vi "UP-COUNTER-V2.vi"() -> (3 "COMPARATOR INPUT 1":u32)   [LabVIEW 2016]
panel:
  in  "LOWER LIMIT":u32=22
  in  "UPPER LIMIT":u32=26
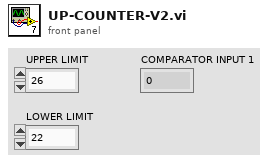
[diagram p1: front panel]
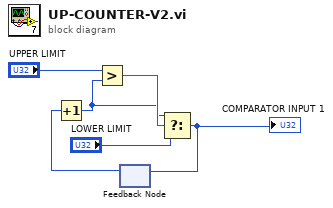
[diagram p0: block diagram]
diagram:
  n1 = feedback #1() -> (w5:u32)  [unwired: 1 in]
  n2 = Increment(x=w5) -> (x+1=w2:u32)
  n3 = Greater?(x="UPPER LIMIT", y=w2) -> (0:w4:bool)
  n4 = Select(t=w2, s=w4, f="LOWER LIMIT") -> (s? t:f=w6:u32)
  "COMPARATOR INPUT 1" <- w6
  n5 = feedback-in #1(w6) -> ()
